vi "TstBldr_Calibration.vi"(0 "Engine reference":refnum<k7>, 2 "m file?":bool, 3 "Paths":T3, 5 "Sequence File Ref":refnum<k7>, 7 "VeriStand version info":T1, 9 "Step Name":string="Open Workspace Manager Reference", 11 "error in":errorcluster, 12 "Conditional Run?":bool, 13 "Sequence index":i32, 14 "Requirement":string) -> (4 "Engine reference (out)":refnum<k7>, 6 "Sequence File Ref(out)":refnum<k7>, 10 "Sequence index (out)":i32, 15 "error out":errorcluster)   [LabVIEW 2010]
doc: "This VI creates the TestStand steps to modify model parameters either by setting multiple parameter values or by updating from a file"
uses:
  FilePaths.ctl
  SeqBuilder/Ctls/dotNetAssemblyInfo.ctl
  SeqBuilder/Ctls/VSModuleTokens.ctl
  vs_SetParamSteps.ctl
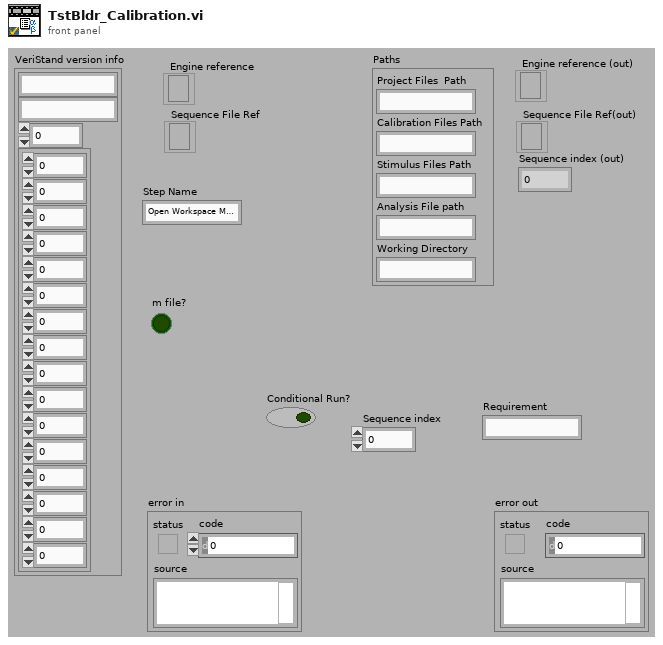
[diagram p1: front panel]
types:
  T1 = typedef "dotNetAssemblyInfo.ctl" = cluster{"VeriStand.exe Path":string, "Assembly":string, "Constructor Token":i32, "Module Token":T2}
  T2 = typedef "VSModuleTokens.ctl" = cluster{"GetIWorkspaceToken":i32, "GetIStimulusToken":i32, "GetIModelManagerToken":i32, "GetIProjectToken":i32, "RunProjectToken":i32, "CloseProjectToken":i32, "RunWorkspaceToken":i32, "StopWorkspaceToken":i32, "SetSingleChannelToken":i32, "SetMultipleParametersToken":i32, "RunStimulusToken":i32, "GetStimulusStateToken":i32, "Open WorkspaceToken":i32, "DeployToken":i32, "UndeployToken":i32, "QuitToken":i32}
  T3 = typedef "FilePaths.ctl" = cluster{"Project Files  Path":string, "Calibration Files Path":string, "Stimulus Files Path":string, "Analysis File path":string, "Working Directory":string}
  T4 = typedef "vs_SetParamSteps.ctl" = enum16{"SetMultipleParam", "Set(m)file", "QuitLoop"}
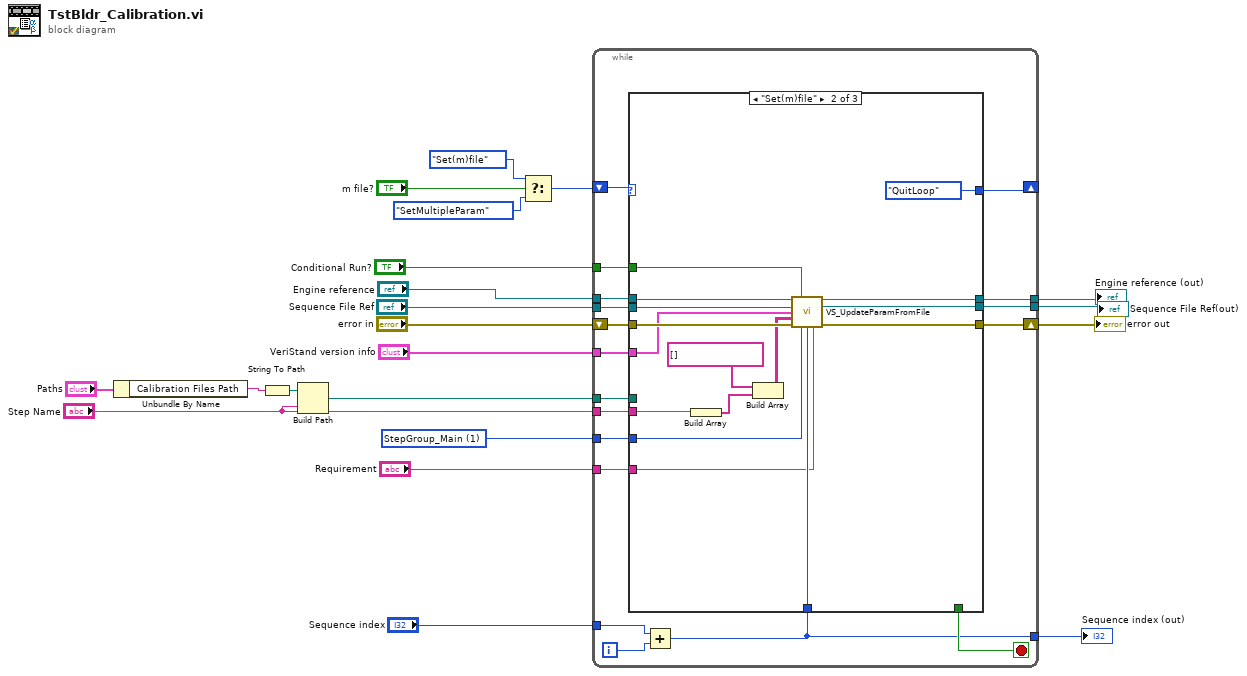
[diagram p0: block diagram]
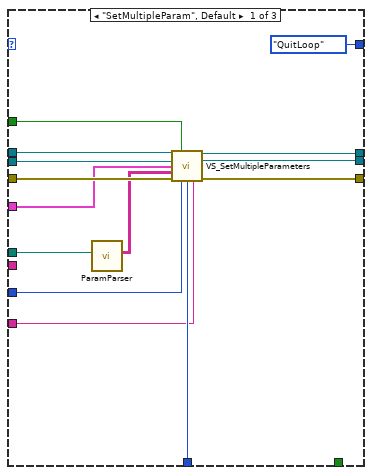
[diagram p2: hidden frame]
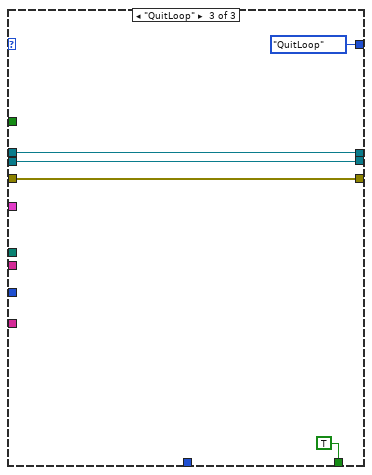
[diagram p3: hidden frame]
diagram:
  w21 = 1 items=["StepGroup_Setup", "StepGroup_Main", "StepGroup_Cleanup"] ("Step Group")
  n1 = Unbundle By Name("Paths") -> ("Calibration Files Path"=w4:string)
  n2 = String To Path(string=w4) -> (path=w2:path)
  n3 = Build Path(base path=w2, name or relative path="Step Name") -> (appended path=w1:path)
  n4 = Select(t=vs_SetParamSteps."Set(m)file" ("Enum"), s="m file?", f=vs_SetParamSteps."SetMultipleParam" ("Enum")) -> (s? t:f=w12:T4)
  n5 = while {
    tunnel: w21 -> [w39]
    tunnel: "Step Name" -> [w38]
    tunnel: "Engine reference" -> [w37]
    tunnel: "Sequence File Ref" -> [w35]
    tunnel: "Sequence index" -> [w29]
    tunnel: "Requirement" -> [w34]
    shift-right: [w32] -> _
    shift-left: w12 -> [w33]
    tunnel: [w28] -> w11
    shift-right: [w27] -> w10
    shift-left: "error in" -> [w36]
    tunnel: "VeriStand version info" -> [w26]
    tunnel: [w25] -> w8
    tunnel: [w24] -> w7
    tunnel: "Conditional Run?" -> [w23]
    tunnel: w1 -> [w22]
    i -> [w30]
    stop <- w31 stop-if-true
    n6 = Add(x=w29, y=w30) -> (x+y=w28:i32)
    n7 = case shown="\"Set(m)file\"" w33 {
      tunnel: w39 -> [w43 w59 _]
      tunnel: w38 -> [_ w56 _]
      tunnel: w37 -> [w48 w65 w72]
      tunnel: w36 -> [w51 w67 w70]
      tunnel: w35 -> [w47 w64 w71]
      tunnel: w34 -> [w42 w58 _]
      tunnel: [vs_SetParamSteps."QuitLoop" ("Enum") vs_SetParamSteps."QuitLoop" ("Enum") vs_SetParamSteps."QuitLoop" ("Enum")] -> w32
      tunnel: [_ _ TRUE] -> w31
      tunnel: w28 -> [w52 w68 _]
      tunnel: [w50 w66 w70] -> w27
      tunnel: w26 -> [w49 w61 _]
      tunnel: [w46 w63 w72] -> w25
      tunnel: [w45 w62 w71] -> w24
      tunnel: w23 -> [w44 w60 _]
      tunnel: w22 -> [w41 _ _]
      frame "SetMultipleParam", Default {
        n8 = call "ParamParser.vi"("Path"=w41) -> ("Calibration values"=w40:string[][])  [unwired: 9 in, 1 out]
        n9 = call "VS_SetMultipleParameters.vi"("Engine Reference(in)"=w48, "Condition Run?"=w44, "Sequence File Ref(in)"=w47, "VeriStand version info"=w49, "Parameter Value array"=w40, "error in"=w51, "Step Group"=w43, "Step Index"=w52, "Requirement"=w42) -> ("Engine reference(out)"=w46:refnum<k7>, "Sequence File Ref(out)"=w45:refnum<k7>, "error out"=w50:errorcluster)  [unwired: 3 in, 1 out]
      }
      frame "Set(m)file" {
        n10 = Build Array(w56) -> (w55:string[])
        n11 = Build Array(string[] [], w55) -> (w54:string[][])
        n12 = call "VS_UpdateParamFromFile.vi"("Engine Reference(in)"=w65, "Condition Run?"=w60, "Sequence File Ref(in)"=w64, "VeriStand version info"=w61, "Parameter Value array"=w54, "error in"=w67, "Step Group"=w59, "Step Index"=w68, "Requirement"=w58) -> ("Engine reference(out)"=w63:refnum<k7>, "Sequence File Ref(out)"=w62:refnum<k7>, "error out"=w66:errorcluster)  [unwired: 3 in, 1 out]
      }
      frame "QuitLoop" {
      }
    }
  }
  "error out" <- w10
  "Sequence File Ref(out)" <- w7
  "Engine reference (out)" <- w8
  "Sequence index (out)" <- w11
